vi "Exp IFaucet Cycling.vi"() -> ()   [LabVIEW 2009]
uses:
  ChannelSettings.ctl
  Intellifaucet/Intellfaucet Mode.ctl
panel:
  out "Numeric":i32
  in  "y":dbl
  in  "milliseconds to wait":u32
  in  "stop":bool
  in  "MW100":refnum<visa-resource-name>
  out "error out":errorcluster
  in  "Semiphore":T1
  in  "error in (no error)":errorcluster
  out "Value":dbl
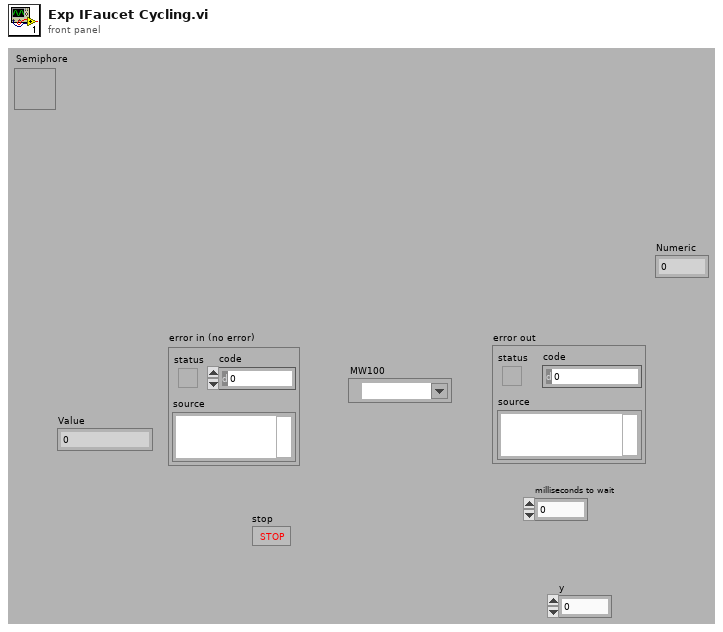
[diagram p1: front panel]
types:
  T1 = typedef "Semaphore RefNum" = refnum<k1>
  T2 = typedef "Intellfaucet Mode.ctl" = enum16{"Adjust Temp", "Adjust Flow", "Start Flow", "Stop Flow"}
  T3 = typedef "ChannelSettings.ctl" = u32
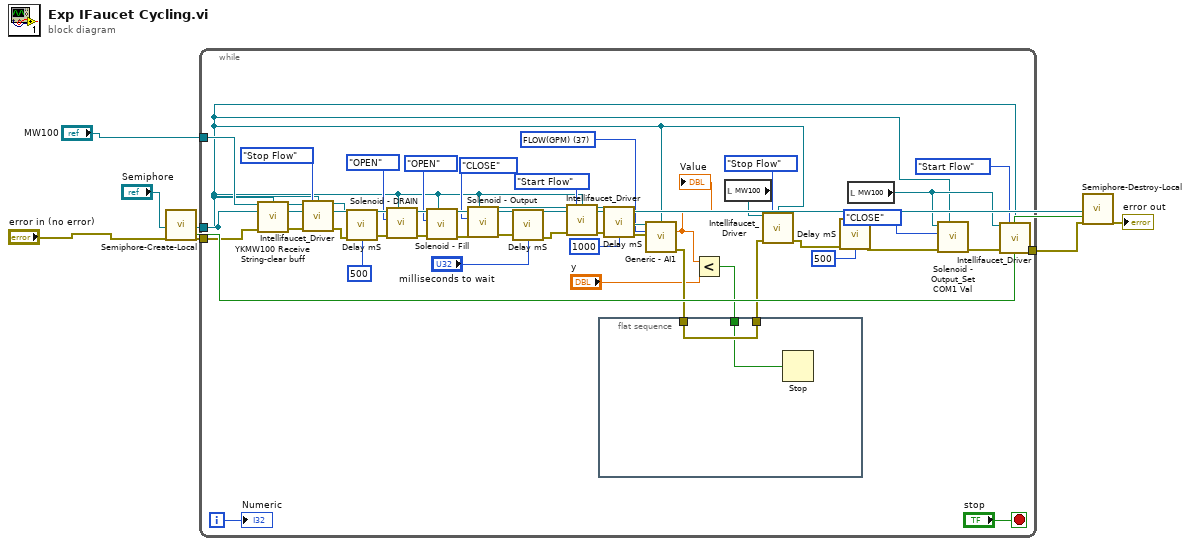
[diagram p0: block diagram]
diagram:
  n1 = call "Semiphore-Create-Local.vi"("Semiphore"="Semiphore", "error in (no error)"="error in (no error)") -> ("semaphore"=w2:T1, "Local?"=w5:bool, "error out"=w6:errorcluster)  [unwired: 15 in]
  n2 = while {
    tunnel: w6 -> [w29]
    tunnel: "MW100" -> [w19]
    tunnel: w2 -> [w15]
    tunnel: [w14] -> w1
    i -> [w9]
    stop <- "stop" stop-if-true
    w36 = T3 37 items=["4-20_OUT", "Pres_HI1", "Pres_HI2", "Pres_LOW", "Pres_PIN", "HEATER_TOP", "HEATER_BOT", "T_Shell", "FLOWMETER", "WATT_SENSE", "WH_TICK", "Tc_1", "Tc_2", "Tc_3", "Tc_4", "Tc_5", "Tc_6", "Tc_down", "T_Shell_2", "T_Shell_3", "T_Shell_4", "RTD_IN", "RTD_OUT", "RTD_AMB", "INTF_TEMPFLO", "INTF_READY", "INTF_START", "INTF_STOP", "DRM_LOW", "DRM_HIGH", "PWR_MAIN", "VLV_DUMP", "VLV_OUT", "VLV_IN", "WATT_HOURS", "FLOW(SAMPLE)", "GALLONS", "FLOW(GPM)"] ("Channel_Enum")
    n3 = call "YKMW100 Receive String-clear buff.vi"("VISA session"=w19, "Semiphore"=w15, "error in (no error)"=w29) -> ("dup VISA session"=w41:refnum<visa-resource-name>, "error out"=w40:errorcluster)  [unwired: 10 in, 1 out]
    n4 = call "Intellifaucet_Driver.vi"("VISA session"=w41, "Mode"=Intellfaucet_Mode."Stop Flow", "Semiphore"=w15, "Error In"=w40) -> ("VISA session out"=w44:refnum<visa-resource-name>, "Error Out"=w43:errorcluster)  [unwired: 10 in]
    n5 = call "Delay mS.vi"("Error In"=w43, "milliseconds to wait"=u32 500) -> ("Error Out"=w42:errorcluster)  [unwired: 13 in]
    n6 = call "Solenoid - DRAIN.vi"("Semiphore"=w15, "Error In"=w42, "VALVE OPEN CLOSE"=enum8{"OPEN", "CLOSE"}."OPEN", "VISA session"=w44) -> ("Error Out"=w52:errorcluster, "dup VISA session"=w51:refnum<visa-resource-name>)  [unwired: 6 in]
    n7 = call "Solenoid - Fill.vi"("Semiphore"=w15, "Error In"=w52, "VALVE OPEN CLOSE"=enum8{"OPEN", "CLOSE"}."OPEN" ("OPEN CLOSE"), "VISA session"=w51) -> ("Error Out"=w49:errorcluster, "dup VISA session"=w48:refnum<visa-resource-name>)  [unwired: 6 in]
    n8 = call "Solenoid - Output.vi"("Semiphore"=w15, "Error In"=w49, "OPEN CLOSE"=enum8{"CLOSE", "OPEN"}."CLOSE", "VISA session"=w48) -> ("Error Out"=w32:errorcluster, "dup VISA session"=w45:refnum<visa-resource-name>)  [unwired: 6 in]
    n9 = call "Delay mS.vi"("Error In"=w32, "milliseconds to wait"="milliseconds to wait") -> ("Error Out"=w31:errorcluster)  [unwired: 13 in]
    n10 = call "Intellifaucet_Driver.vi"("VISA session"=w45, "Mode"=Intellfaucet_Mode."Start Flow", "Semiphore"=w15, "Error In"=w31) -> ("VISA session out"=w37:refnum<visa-resource-name>, "Error Out"=w39:errorcluster)  [unwired: 10 in]
    n11 = flat-sequence {
      tunnel: [w54] -> w18
      tunnel: w17 -> [w54]
      tunnel: w10 -> [w53]
      frame #0 {
        n12 = Stop(stop? (T)=w53) -> ()
      }
    }
    n13 = call "Delay mS.vi"("Error In"=w39, "milliseconds to wait"=u32 1000) -> ("Error Out"=w38:errorcluster)  [unwired: 13 in]
    n14 = call "Generic - AI1.vi"("MW100"=w37, "Semiphore"=w15, "Channel_Enum"=w36, "Error In"=w38) -> ("Value"=w12:dbl, "Error Out"=w17:errorcluster)  [unwired: 9 in, 1 out]
    "Value" <- w12
    n15 = Less?(x=w12, y="y") -> (x < y?=w10:bool)
    n16 = local read "MW100"() -> (w21:refnum<visa-resource-name>)
    n17 = call "Intellifaucet_Driver.vi"("VISA session"=w21, "Mode"=Intellfaucet_Mode."Stop Flow", "Semiphore"=w15, "Error In"=w18) -> ("Error Out"=w22:errorcluster)  [unwired: 10 in, 1 out]
    n18 = call "Delay mS.vi"("Error In"=w22, "milliseconds to wait"=u32 500) -> ("Error Out"=w23:errorcluster)  [unwired: 13 in]
    n19 = local read "MW100"() -> (w26:refnum<visa-resource-name>)
    n20 = call "Solenoid - Output_Set COM1 Val.vi"("Semiphore"=w15, "Error In"=w23, "OPEN CLOSE"=enum8{"CLOSE", "OPEN"}."CLOSE", "VISA session"=w26) -> ("Error Out"=w25:errorcluster)  [unwired: 6 in, 1 out]
    n21 = call "Intellifaucet_Driver.vi"("VISA session"=w26, "Mode"=Intellfaucet_Mode."Start Flow", "Semiphore"=w15, "Error In"=w25) -> ("Error Out"=w14:errorcluster)  [unwired: 10 in, 1 out]
    "Numeric" <- w9
  }
  n22 = call "Semiphore-Destroy-Local.vi"("Semiphore"=w2, "Local?"=w5, "error in (no error)"=w1) -> ("error out"=→"error out":errorcluster)  [unwired: 16 in]
